vi "Reset N attempt.vi"(8 "error in (no error)":errorcluster, 11 "MB_TCP in":refnum<class "MB_TCP.lvclass">) -> (0 "error out":errorcluster, 3 "MB_TCP out":refnum<class "MB_TCP.lvclass">)   [LabVIEW 2021, in "MB_TCP.lvclass"]
uses:
  MB_TCP.lvclass
  MB_TCP.lvclass/MB_TCP.ctl
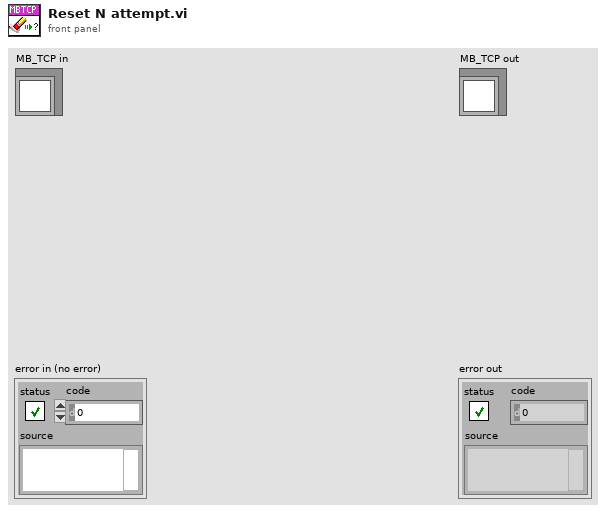
[diagram p1: front panel]
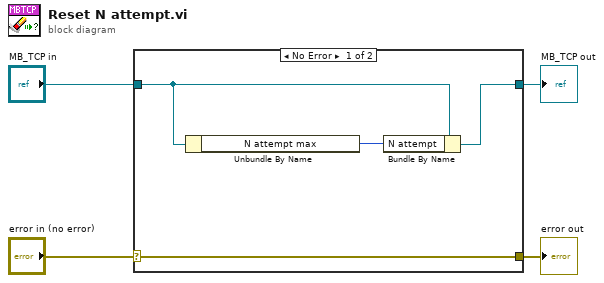
[diagram p0: block diagram]
diagram:
  n1 = case shown="No Error" "error in (no error)" {
    selector: "error in (no error)" -> [w8 w9]
    tunnel: [w8 w9] -> w3
    tunnel: [w7 w10] -> w1
    tunnel: "MB_TCP in" -> [w6 w10]
    frame No Error {
      n2 = Unbundle By Name(w6) -> ("N attempt max"=w5:i32)
      n3 = Bundle By Name(cluster=w6, "N attempt"=w5) -> (w7:refnum<class "MB_TCP.lvclass">)
    }
    frame Error {
    }
  }
  "error out" <- w3
  "MB_TCP out" <- w1
